vi "from string.vi"(8 "error in":errorcluster, 9 "data":string, 10 "version":string, 11 "SystemLin Tag Module configuration in":refnum<class "SystemLink configuration.lvclass">) -> (0 "error out":errorcluster, 3 "SystemLin Tag Module configuration out":refnum<class "SystemLink configuration.lvclass">)   [LabVIEW 2015, in "SystemLink configuration.lvclass"]
doc: "Provides an interface for loading a module configuration from a file or other serialized data source. It is recommended that all children of this class store data in two sets--data required for its own initialization, and any data required for parent initialization--and that each implementation uses the <b>Call Parent Method</b> primitive to de-serialize parent information. As a result, it is expected that every module configuration class calls <b>component configuration.lvclass:From String.vi</b>."
uses:
  SystemLink configuration.lvclass
  <vilib>/NI/Tag Bus Module Framework/channel/TBM channel.lvclass
  Line.ctl
  Data Tag Type.ctl
  SystemLink configuration.lvclass/SystemLink configuration.ctl
  <vilib>/NI/Tag Bus Module Framework/module configuration/TBM module configuration.lvclass
  <vilib>/NI/Configuration Framework/serializable configuration/NISE_CEF_serializable configuration.lvclass
  <vilib>/NI/Tag Bus/tag/tag descriptor.lvclass
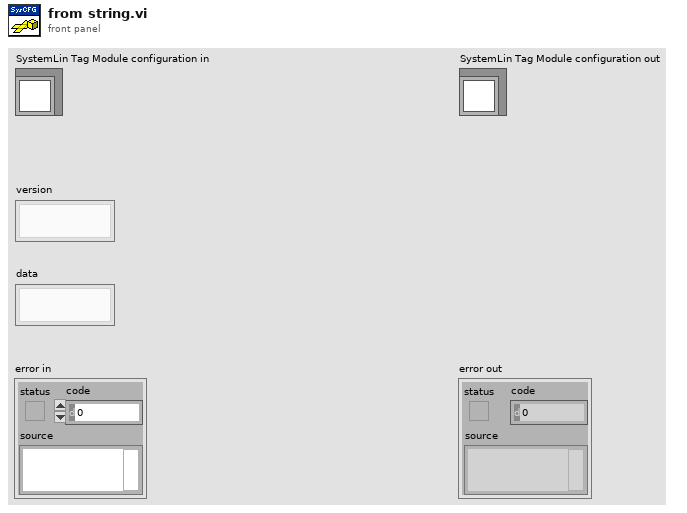
[diagram p1: front panel]
types:
  T1 = enum16{"Double", "Single", "I32", "I16", "I8", "U64", "U32", "U16", "U8", "Boolean", "String", "Timestamp"}
  T2 = typedef "SystemLink configuration.lvclass/Line.ctl" = cluster{"channel":refnum<class "TBM channel.lvclass">, "Data Tag Type":T3}
  T3 = typedef "SystemLink configuration.lvclass/Data Tag Type.ctl" = enum16{"Double", "Single", "I32", "I16", "I8", "U64", "U32", "U16", "U8", "Boolean", "String", "Timestamp"}
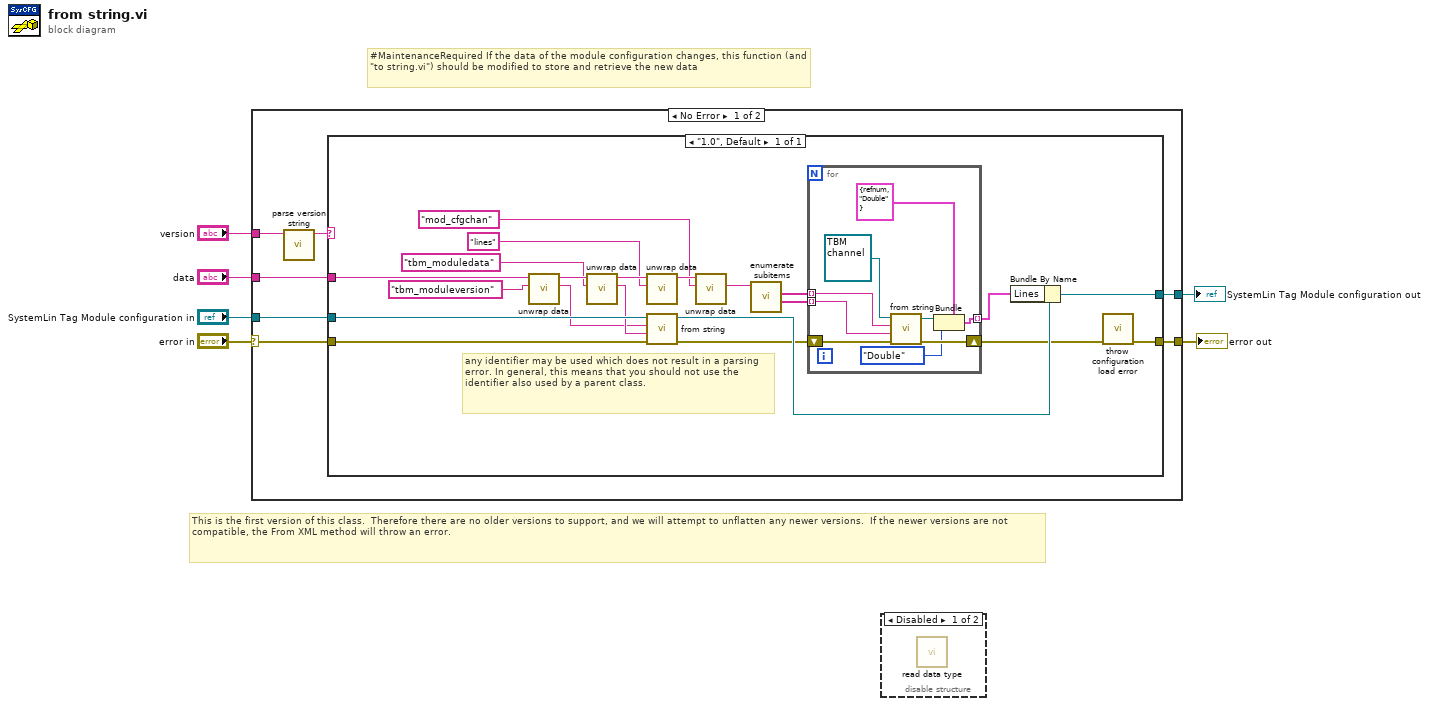
[diagram p0: block diagram]
diagram:
  # "#MaintenanceRequired If the data of the module configuration changes, this function (and \"to string.vi\") should be modified to store and retrieve the new data"
  # "This is the first version of this class.  Therefore there are no older versions to support, and we will attempt to unflatten any newer versions.  If the newer versions are not compatible, the From XML method will throw an error."
  n1 = case shown="No Error" "error in" {
    selector: "error in" -> [w7 w45]
    tunnel: "data" -> [w13 _]
    tunnel: "SystemLin Tag Module configuration in" -> [w12 w44]
    tunnel: [w11 w44] -> w5
    tunnel: [w10 w45] -> w4
    tunnel: "version" -> [w9 _]
    frame No Error {
      n2 = call <vilib>:"parse version string.vi"("full version"=w9) -> ("major.minor version"=w8:string)  [unwired: 7 in, 3 out]
      n3 = case shown="\"1.0\", Default" w8 {
        tunnel: w13 -> [w31]
        tunnel: w7 -> [w30]
        tunnel: w12 -> [w34]
        tunnel: [w22] -> w11
        tunnel: [w33] -> w10
        frame "1.0", Default {
          # "any identifier may be used which does not result in a parsing error. In general, this means that you should not use the identifier also used by a parent class."
          n4 = call <vilib>:"unwrap data.vi"("identifier"="tbm_moduleversion" ("additional identifier"), "data to unwrap"=w31) -> ("unwrapped data"=w26:string, "remaining string"=w32:string)  [unwired: 8 in]
          n5 = call <vilib>:"unwrap data.vi"("identifier"="tbm_moduledata" ("additional identifier"), "data to unwrap"=w32) -> ("unwrapped data"=w28:string, "remaining string"=w25:string)  [unwired: 8 in]
          n6 = call <vilib>:"unwrap data.vi"("identifier"="lines" ("additional identifier"), "data to unwrap"=w25) -> ("remaining string"=w21:string)  [unwired: 8 in, 1 out]
          n7 = call-parent "from string.vi"("error in"=w30, "data"=w28, "version"=w26, "module configuration in"=w34) -> ("error out"=w17:errorcluster, "module configuration out"=w23:refnum<class "SystemLink configuration.lvclass">)  [unwired: 6 in]
          n8 = call <vilib>:"unwrap data.vi"("identifier"="mod_cfgchan", "data to unwrap"=w21) -> ("unwrapped data"=w16:string)  [unwired: 8 in, 1 out]
          n9 = call <vilib>:"enumerate subitems.vi"("data to enumerate"=w16) -> ("associated data"=w18:string[], "discovered subitems"=w19:string[])  [unwired: 8 in, 1 out]
          n10 = for {
            shift-right: [w43] -> w14
            shift-left: w17 -> [w42]
            tunnel: w19 -> [w41] mode=indexing
            tunnel: w18 -> [w40] mode=indexing
            tunnel: [w36] -> w15 mode=indexing
            n11 = call-dynamic "from string.vi"("error in"=w42, "channel data"=w40, "identifier"=w41, "channel in"=refnum<class "TBM channel.lvclass"> refnum) -> ("error out"=w43:errorcluster, "channel out"=w37:refnum<class "TBM channel.lvclass">)  [unwired: 6 in]
            n12 = Bundle(cluster=T2 {"channel"=refnum, "Data Tag Type"=enum."Double"} ("Line"), "channel"=w37, "Data Tag Type"=T1."Double") -> (w36:T2)
          }
          n13 = Bundle By Name(cluster=w23, "Lines"=w15) -> (w22:refnum<class "SystemLink configuration.lvclass">)
          n14 = call <vilib>:"throw configuration load error.vi"("error in"=w14) -> ("error out"=w33:errorcluster)  [unwired: 10 in]
        }
      }
    }
    frame Error {
    }
  }
  "error out" <- w4
  "SystemLin Tag Module configuration out" <- w5
  n15 = disable-structure shown="Disabled" {
    frame Disabled {
      n16 = call <vilib>:"read data type.vi"() -> ()  [unwired: 9 in, 3 out]
    }
    frame Enabled {
    }
  }
